vi "Start Sync.vi"(8 "error in (no error)":errorcluster, 11 "gRPC Server in":refnum<class "NiDAQmx.lvclass">) -> (0 "error out":errorcluster, 3 "gRPC Server out":refnum<class "NiDAQmx.lvclass">)   [LabVIEW 2021, in "NI DAQmx_server.lvlib" / "NiDAQmx.lvclass"]
uses:
  NiDAQmx.lvclass
  NiDAQmx.lvclass/NiDAQmx.ctl
  NI DAQmx_wrapper/NI DAQmx_wrapper.lvlib
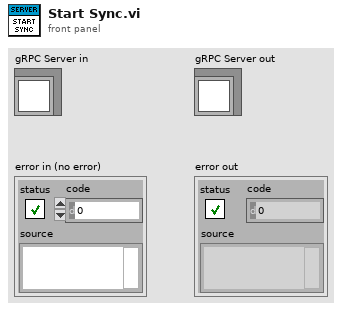
[diagram p1: front panel]
types:
  T1 = typedef "NI DAQmx_server.lvlib/NiDAQmx.lvclass/Server Internal UEs.ctl" = cluster{"NiDAQmx CreateTask Internal UE":refnum<user-event>, "NiDAQmx CreateDOChan Internal UE":refnum<user-event>, "NiDAQmx CreateCIFreqChan Internal UE":refnum<user-event>, "NiDAQmx WriteDigitalLines Internal UE":refnum<user-event>, "NiDAQmx ReadCounterScalarF64 Internal UE":refnum<user-event>, "NiDAQmx CfgImplicitTiming Internal UE":refnum<user-event>, "NiDAQmx StartTask Internal UE":refnum<user-event>, "NiDAQmx StopTask Internal UE":refnum<user-event>, "NiDAQmx ClearTask Internal UE":refnum<user-event>, "NiDAQmx GetTaskAttributeString Internal UE":refnum<user-event>, "NiDAQmx GetChanAttributeString Internal UE":refnum<user-event>, "NiDAQmx GetChanAttributeDouble Internal UE":refnum<user-event>, "NiDAQmx SetChanAttributeString Internal UE":refnum<user-event>, "NiDAQmx SetChanAttributeDouble Internal UE":refnum<user-event>}
  T2 = typedef "NI DAQmx_server.lvlib/NiDAQmx.lvclass/Server gRPC UEs.ctl" = cluster{"NiDAQmx CreateTask gRPC UE":refnum<user-event>, "NiDAQmx CreateDOChan gRPC UE":refnum<user-event>, "NiDAQmx CreateCIFreqChan gRPC UE":refnum<user-event>, "NiDAQmx WriteDigitalLines gRPC UE":refnum<user-event>, "NiDAQmx ReadCounterScalarF64 gRPC UE":refnum<user-event>, "NiDAQmx CfgImplicitTiming gRPC UE":refnum<user-event>, "NiDAQmx StartTask gRPC UE":refnum<user-event>, "NiDAQmx StopTask gRPC UE":refnum<user-event>, "NiDAQmx ClearTask gRPC UE":refnum<user-event>, "NiDAQmx GetTaskAttributeString gRPC UE":refnum<user-event>, "NiDAQmx GetChanAttributeString gRPC UE":refnum<user-event>, "NiDAQmx GetChanAttributeDouble gRPC UE":refnum<user-event>, "NiDAQmx SetChanAttributeString gRPC UE":refnum<user-event>, "NiDAQmx SetChanAttributeDouble gRPC UE":refnum<user-event>}
  T3 = typedef "grpc-lvsupport-release.lvlib/grpcId.ctl" = u64
  T4 = typedef "NI DAQmx_server.lvlib/nidaqmx_grpc_CreateTaskRequest.ctl" = cluster{"session_name":string, "initialization_behavior":T5}
  T5 = typedef "NI DAQmx_server.lvlib/nidevice_grpc_SessionInitializationBehavior.ctl" = enum32{"SESSION_INITIALIZATION_BEHAVIOR_UNSPECIFIED", "SESSION_INITIALIZATION_BEHAVIOR_INITIALIZE_NEW", "SESSION_INITIALIZATION_BEHAVIOR_ATTACH_TO_EXISTING"}
  T6 = typedef "NI DAQmx_server.lvlib/nidaqmx_grpc_CreateTaskResponse.ctl" = cluster{"status":i32, "task":T7, "new_session_initialized":bool}
  T7 = typedef "NI DAQmx_server.lvlib/nidevice_grpc_Session.ctl" = cluster{"nidevice_grpc_Session_session":refnum<class "nidevice_grpc_Session_session.lvclass">}
  T8 = typedef "NI DAQmx_server.lvlib/nidaqmx_grpc_CreateDOChanRequest.ctl" = cluster{"task":T7, "lines":string, "name_to_assign_to_lines":string, "nidaqmx_grpc_CreateDOChanRequest_line_grouping_enum":refnum<class "nidaqmx_grpc_CreateDOChanRequest_line_grouping_enum.lvclass">}
  T9 = typedef "NI DAQmx_server.lvlib/nidaqmx_grpc_CreateDOChanResponse.ctl" = cluster{"status":i32}
  T10 = typedef "NI DAQmx_server.lvlib/nidaqmx_grpc_CreateCIFreqChanRequest.ctl" = cluster{"task":T7, "counter":string, "name_to_assign_to_channel":string, "min_val":dbl, "max_val":dbl, "nidaqmx_grpc_CreateCIFreqChanRequest_units_enum":refnum<class "nidaqmx_grpc_CreateCIFreqChanRequest_units_enum.lvclass">, "nidaqmx_grpc_CreateCIFreqChanRequest_edge_enum":refnum<class "nidaqmx_grpc_CreateCIFreqChanRequest_edge_enum.lvclass">, "nidaqmx_grpc_CreateCIFreqChanRequest_meas_method_enum":refnum<class "nidaqmx_grpc_CreateCIFreqChanRequest_meas_method_enum.lvclass">, "meas_time":dbl, "divisor":u32, "custom_scale_name":string}
  T11 = typedef "NI DAQmx_server.lvlib/nidaqmx_grpc_CreateCIFreqChanResponse.ctl" = cluster{"status":i32}
  T12 = typedef "NI DAQmx_server.lvlib/nidaqmx_grpc_WriteDigitalLinesRequest.ctl" = cluster{"task":T7, "num_samps_per_chan":i32, "auto_start":bool, "timeout":dbl, "nidaqmx_grpc_WriteDigitalLinesRequest_data_layout_enum":refnum<class "nidaqmx_grpc_WriteDigitalLinesRequest_data_layout_enum.lvclass">, "write_array":u8[]}
  T13 = typedef "NI DAQmx_server.lvlib/nidaqmx_grpc_WriteDigitalLinesResponse.ctl" = cluster{"status":i32, "samps_per_chan_written":i32}
  T14 = typedef "NI DAQmx_server.lvlib/nidaqmx_grpc_ReadCounterScalarF64Request.ctl" = cluster{"task":T7, "timeout":dbl}
  T15 = typedef "NI DAQmx_server.lvlib/nidaqmx_grpc_ReadCounterScalarF64Response.ctl" = cluster{"status":i32, "value":dbl}
  T16 = typedef "NI DAQmx_server.lvlib/nidaqmx_grpc_CfgImplicitTimingRequest.ctl" = cluster{"task":T7, "nidaqmx_grpc_CfgImplicitTimingRequest_sample_mode_enum":refnum<class "nidaqmx_grpc_CfgImplicitTimingRequest_sample_mode_enum.lvclass">, "samps_per_chan":u64}
  T17 = typedef "NI DAQmx_server.lvlib/nidaqmx_grpc_CfgImplicitTimingResponse.ctl" = cluster{"status":i32}
  T18 = typedef "NI DAQmx_server.lvlib/nidaqmx_grpc_StartTaskRequest.ctl" = cluster{"task":T7}
  T19 = typedef "NI DAQmx_server.lvlib/nidaqmx_grpc_StartTaskResponse.ctl" = cluster{"status":i32}
  T20 = typedef "NI DAQmx_server.lvlib/nidaqmx_grpc_StopTaskRequest.ctl" = cluster{"task":T7}
  T21 = typedef "NI DAQmx_server.lvlib/nidaqmx_grpc_StopTaskResponse.ctl" = cluster{"status":i32}
  T22 = typedef "NI DAQmx_server.lvlib/nidaqmx_grpc_ClearTaskRequest.ctl" = cluster{"task":T7}
  T23 = typedef "NI DAQmx_server.lvlib/nidaqmx_grpc_ClearTaskResponse.ctl" = cluster{"status":i32}
  T24 = typedef "NI DAQmx_server.lvlib/nidaqmx_grpc_GetTaskAttributeStringRequest.ctl" = cluster{"task":T7, "nidaqmx_grpc_GetTaskAttributeStringRequest_attribute_enum":refnum<class "nidaqmx_grpc_GetTaskAttributeStringRequest_attribute_enum.lvclass">}
  T25 = typedef "NI DAQmx_server.lvlib/nidaqmx_grpc_GetTaskAttributeStringResponse.ctl" = cluster{"status":i32, "value":string}
  T26 = typedef "NI DAQmx_server.lvlib/nidaqmx_grpc_GetChanAttributeStringRequest.ctl" = cluster{"task":T7, "channel":string, "nidaqmx_grpc_GetChanAttributeStringRequest_attribute_enum":refnum<class "nidaqmx_grpc_GetChanAttributeStringRequest_attribute_enum.lvclass">}
  T27 = typedef "NI DAQmx_server.lvlib/nidaqmx_grpc_GetChanAttributeStringResponse.ctl" = cluster{"status":i32, "value":string}
  T28 = typedef "NI DAQmx_server.lvlib/nidaqmx_grpc_GetChanAttributeDoubleRequest.ctl" = cluster{"task":T7, "channel":string, "nidaqmx_grpc_GetChanAttributeDoubleRequest_attribute_enum":refnum<class "nidaqmx_grpc_GetChanAttributeDoubleRequest_attribute_enum.lvclass">}
  T29 = typedef "NI DAQmx_server.lvlib/nidaqmx_grpc_GetChanAttributeDoubleResponse.ctl" = cluster{"status":i32, "value":dbl}
  T30 = typedef "NI DAQmx_server.lvlib/nidaqmx_grpc_SetChanAttributeStringRequest.ctl" = cluster{"task":T7, "channel":string, "nidaqmx_grpc_SetChanAttributeStringRequest_attribute_enum":refnum<class "nidaqmx_grpc_SetChanAttributeStringRequest_attribute_enum.lvclass">, "value":string}
  T31 = typedef "NI DAQmx_server.lvlib/nidaqmx_grpc_SetChanAttributeStringResponse.ctl" = cluster{"status":i32}
  T32 = typedef "NI DAQmx_server.lvlib/nidaqmx_grpc_SetChanAttributeDoubleRequest.ctl" = cluster{"task":T7, "channel":string, "nidaqmx_grpc_SetChanAttributeDoubleRequest_attribute_enum":refnum<class "nidaqmx_grpc_SetChanAttributeDoubleRequest_attribute_enum.lvclass">, "value":dbl}
  T33 = typedef "NI DAQmx_server.lvlib/nidaqmx_grpc_SetChanAttributeDoubleResponse.ctl" = cluster{"status":i32}
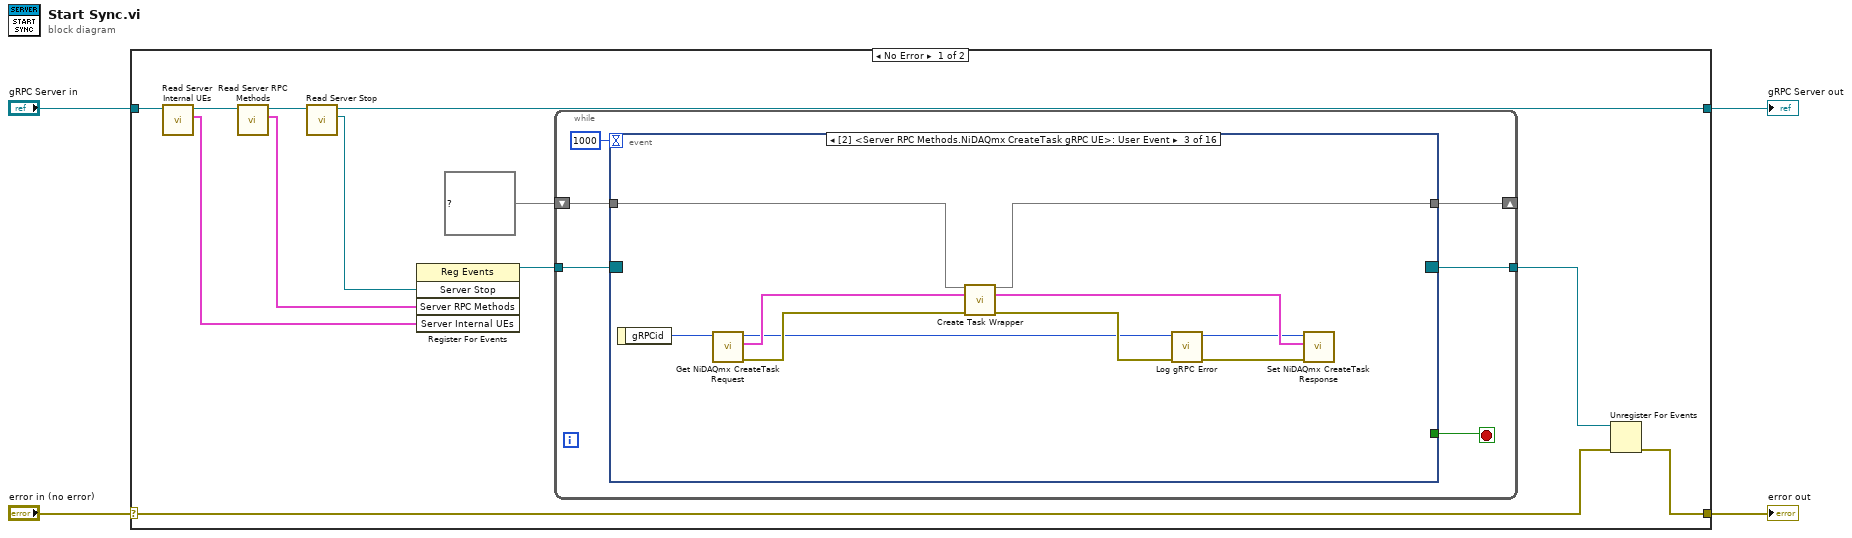
[diagram p0: block diagram]
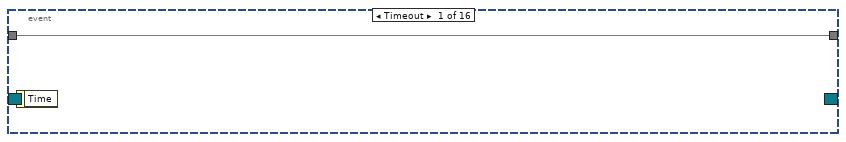
[diagram p2: hidden frame]
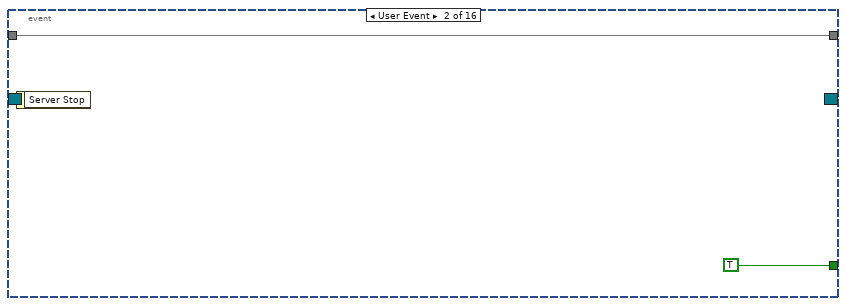
[diagram p3: hidden frame]
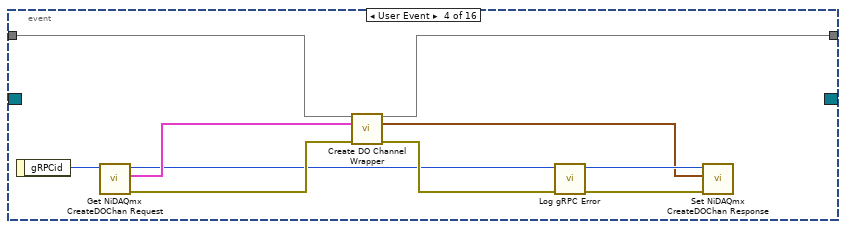
[diagram p4: hidden frame]
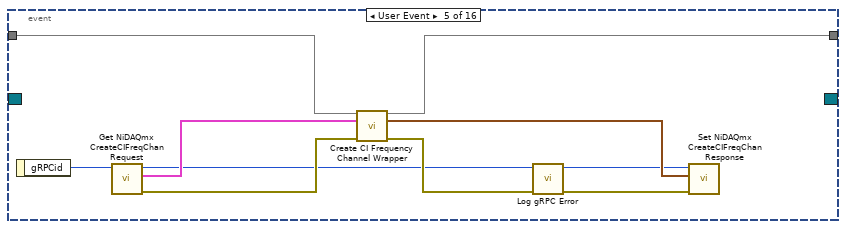
[diagram p5: hidden frame]
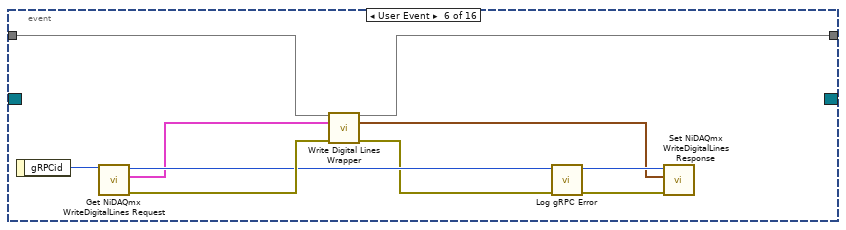
[diagram p6: hidden frame]
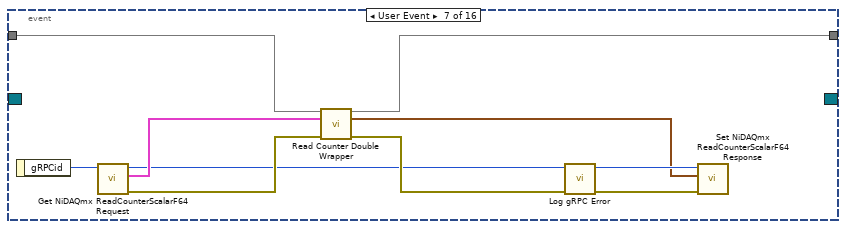
[diagram p7: hidden frame]
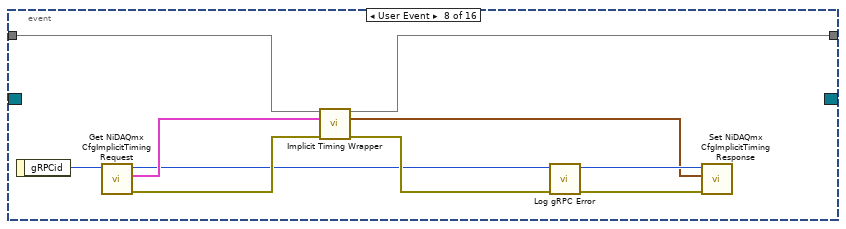
[diagram p8: hidden frame]
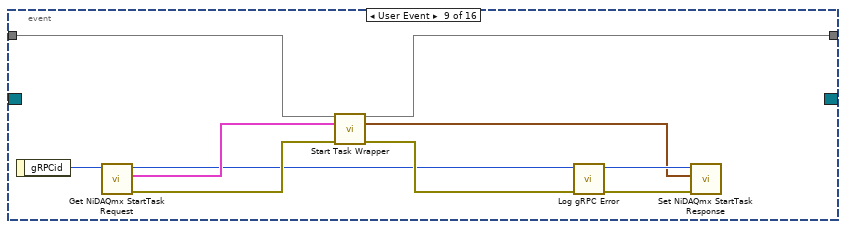
[diagram p9: hidden frame]
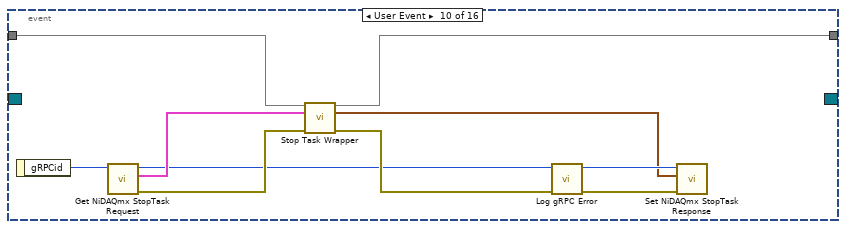
[diagram p10: hidden frame]
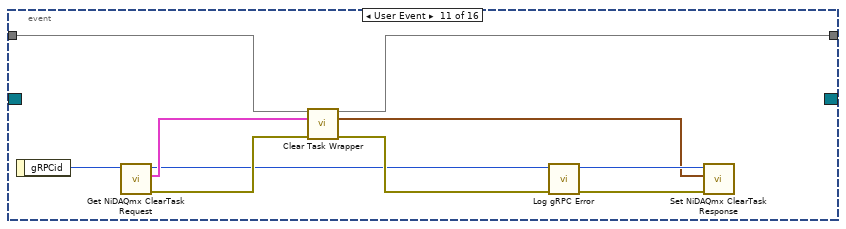
[diagram p11: hidden frame]
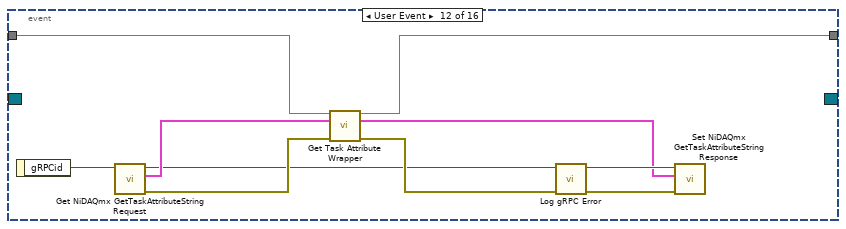
[diagram p12: hidden frame]
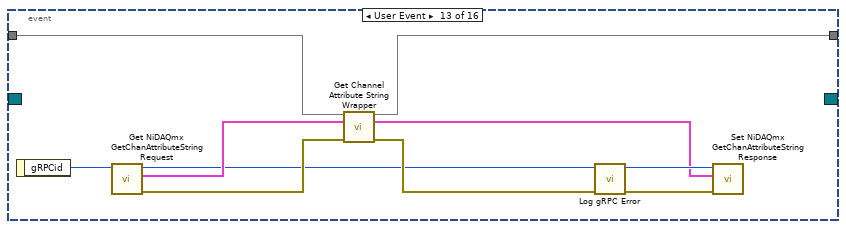
[diagram p13: hidden frame]
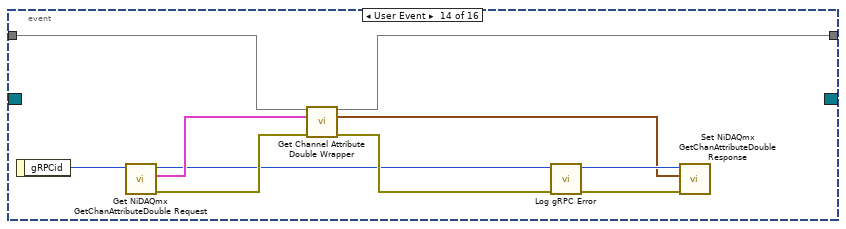
[diagram p14: hidden frame]
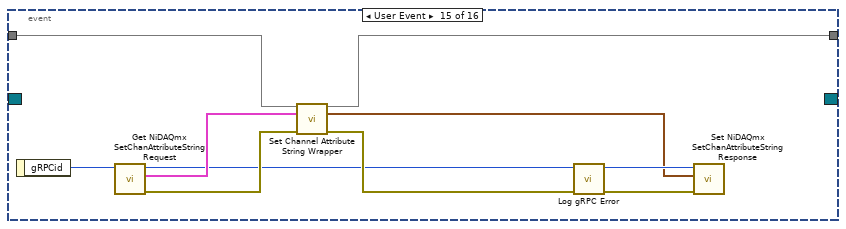
[diagram p15: hidden frame]
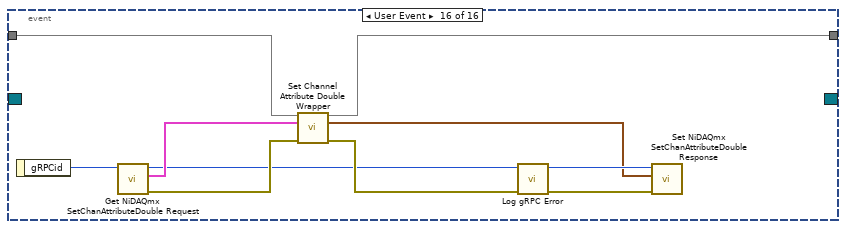
[diagram p16: hidden frame]
diagram:
  n1 = case shown="No Error" "error in (no error)" {
    selector: "error in (no error)" -> [w10 w167]
    tunnel: [w9 w167] -> w3
    tunnel: [w7 w166] -> w1
    tunnel: "gRPC Server in" -> [w16 w166]
    frame No Error {
      n2 = call "Read Server Internal UEs.vi"("SignalGeneratorService in"=w16) -> ("Server Internal UEs"=w14:T1, "SignalGeneratorService out"=w15:refnum<class "NiDAQmx.lvclass">)  [unwired: 8 in, 1 out]
      n3 = call "Read Server RPC Methods.vi"("SignalGeneratorService in"=w15) -> ("Server RPC Methods"=w8:T2, "SignalGeneratorService out"=w13:refnum<class "NiDAQmx.lvclass">)  [unwired: 8 in, 1 out]
      n4 = call-dynamic "Read Server Stop.vi"("iService in"=w13) -> ("Server Stop"=w6:refnum<user-event>, "iService out"=w7:refnum<class "NiDAQmx.lvclass">)  [unwired: 8 in, 1 out]
      n5 = register-events(w6, w8, w14) -> (reference out=w12:refnum<event-registration>)  [unwired: 2 in, 1 out]
      n6 = while {
        tunnel: w12 -> [w22]
        tunnel: [w20] -> w11
        shift-right: [w17] -> _
        shift-left: map{string, refnum<k21>} {} ("Task map") -> [w18]
        stop <- w21 stop-if-true
        n7 = event "RPC Methods Event Structure" shown="[2] <Server RPC Methods.NiDAQmx CreateTask gRPC UE>: User Event" {
          selector: w22 -> [_ _ _ _ _ _ _ _ _ _ _ _ _ _ _ _]
          dyn-events: [_ _ _ _ _ _ _ _ _ _ _ _ _ _ _ _] -> w20
          timeout: 1000 -> [_ _ _ _ _ _ _ _ _ _ _ _ _ _ _ _]
          tunnel: [_ TRUE _ _ _ _ _ _ _ _ _ _ _ _ _ _] -> w21
          tunnel: w18 -> [w23 w24 w32 w42 w47 w60 w73 w82 w92 w102 w113 w123 w132 w142 w152 w162]
          tunnel: [w23 w24 w30 w36 w46 w58 w71 w77 w91 w100 w107 w116 w127 w137 w150 w157] -> w17
          event Timeout {
            n8 = event-data() -> ()  [unwired: 1 in, 1 out]
          }
          event User Event {
            n9 = event-data() -> ()  [unwired: 1 in, 1 out]
          }
          event User Event {
            n10 = event-data() -> ("gRPCid"=w35:T3)  [unwired: 1 in]
            n11 = call "Get NiDAQmx CreateTask Request.vi"("gRPCid"=w35) -> ("error out"=w34:errorcluster, "Message Data"=w33:T4, "gRPCid out"=w27:T3)  [unwired: 8 in]
            n12 = call "Create Task Wrapper.vi"("Task map in"=w32, "Message Data in"=w33, "error in (no error)"=w34) -> ("Task map out"=w30:map{string, refnum<k21>}, "Message Data out"=w31:T6, "error out"=w29:errorcluster)  [unwired: 10 in]
            n13 = call "Log gRPC Error.vi"("error IO"=w29, "gRPC ID in"=w27) -> ("error out"=w28:errorcluster, "gRPCid out"=w26:T3)  [unwired: 8 in]
            n14 = call "Set NiDAQmx CreateTask Response.vi"("error in (no error)"=w28, "Message Data"=w31, "gRPCid in"=w26) -> ()  [unwired: 8 in, 1 out]
          }
          event User Event {
            n15 = event-data() -> ("gRPCid"=w45:T3)  [unwired: 1 in]
            n16 = call "Get NiDAQmx CreateDOChan Request.vi"("gRPCid"=w45) -> ("error out"=w44:errorcluster, "Message Data"=w43:T8, "gRPCid out"=w39:T3)  [unwired: 8 in]
            n17 = call "Create DO Channel Wrapper.vi"("Task map in"=w42, "Message Data in"=w43, "error in (no error)"=w44) -> ("Task map out"=w36:map{string, refnum<k21>}, "Message Data out"=w37:T9, "error out"=w41:errorcluster)  [unwired: 10 in]
            n18 = call "Log gRPC Error.vi"("error IO"=w41, "gRPC ID in"=w39) -> ("error out"=w40:errorcluster, "gRPCid out"=w38:T3)  [unwired: 8 in]
            n19 = call "Set NiDAQmx CreateDOChan Response.vi"("error in (no error)"=w40, "Message Data"=w37, "gRPCid in"=w38) -> ()  [unwired: 8 in, 1 out]
          }
          event User Event {
            n20 = event-data() -> ("gRPCid"=w55:T3)  [unwired: 1 in]
            n21 = call "Get NiDAQmx CreateCIFreqChan Request.vi"("gRPCid"=w55) -> ("error out"=w54:errorcluster, "Message Data"=w53:T10, "gRPCid out"=w49:T3)  [unwired: 8 in]
            n22 = call "Create CI Frequency Channel Wrapper.vi"("Task map in"=w47, "Message Data in"=w53, "error in (no error)"=w54) -> ("Task map out"=w46:map{string, refnum<k21>}, "Message Data out"=w50:T11, "error out"=w51:errorcluster)  [unwired: 10 in]
            n23 = call "Log gRPC Error.vi"("error IO"=w51, "gRPC ID in"=w49) -> ("error out"=w52:errorcluster, "gRPCid out"=w48:T3)  [unwired: 8 in]
            n24 = call "Set NiDAQmx CreateCIFreqChan Response.vi"("error in (no error)"=w52, "Message Data"=w50, "gRPCid in"=w48) -> ()  [unwired: 8 in, 1 out]
          }
          event User Event {
            n25 = event-data() -> ("gRPCid"=w65:T3)  [unwired: 1 in]
            n26 = call "Get NiDAQmx WriteDigitalLines Request.vi"("gRPCid"=w65) -> ("error out"=w64:errorcluster, "Message Data"=w59:T12, "gRPCid out"=w62:T3)  [unwired: 8 in]
            n27 = call "Write Digital Lines Wrapper.vi"("Task map in"=w60, "Message Data in"=w59, "error in (no error)"=w64) -> ("Task map out"=w58:map{string, refnum<k21>}, "Message Data out"=w57:T13, "error out"=w56:errorcluster)  [unwired: 10 in]
            n28 = call "Log gRPC Error.vi"("error IO"=w56, "gRPC ID in"=w62) -> ("error out"=w63:errorcluster, "gRPCid out"=w61:T3)  [unwired: 8 in]
            n29 = call "Set NiDAQmx WriteDigitalLines Response.vi"("error in (no error)"=w63, "Message Data"=w57, "gRPCid in"=w61) -> ()  [unwired: 8 in, 1 out]
          }
          event User Event {
            n30 = event-data() -> ("gRPCid"=w75:T3)  [unwired: 1 in]
            n31 = call "Get NiDAQmx ReadCounterScalarF64 Request.vi"("gRPCid"=w75) -> ("error out"=w74:errorcluster, "Message Data"=w72:T14, "gRPCid out"=w68:T3)  [unwired: 8 in]
            n32 = call "Read Counter Double Wrapper.vi"("Task map in"=w73, "Message Data in"=w72, "error in (no error)"=w74) -> ("Task map out"=w71:map{string, refnum<k21>}, "Message Data Out"=w66:T15, "error out"=w70:errorcluster)  [unwired: 10 in]
            n33 = call "Log gRPC Error.vi"("error IO"=w70, "gRPC ID in"=w68) -> ("error out"=w69:errorcluster, "gRPCid out"=w67:T3)  [unwired: 8 in]
            n34 = call "Set NiDAQmx ReadCounterScalarF64 Response.vi"("error in (no error)"=w69, "Message Data"=w66, "gRPCid in"=w67) -> ()  [unwired: 8 in, 1 out]
          }
          event User Event {
            n35 = event-data() -> ("gRPCid"=w85:T3)  [unwired: 1 in]
            n36 = call "Get NiDAQmx CfgImplicitTiming Request.vi"("gRPCid"=w85) -> ("error out"=w84:errorcluster, "Message Data"=w83:T16, "gRPCid out"=w79:T3)  [unwired: 8 in]
            n37 = call "Implicit Timing Wrapper.vi"("Task map in"=w82, "Message Data in"=w83, "error in (no error)"=w84) -> ("Task map out"=w77:map{string, refnum<k21>}, "Message Data out"=w76:T17, "error out"=w81:errorcluster)  [unwired: 10 in]
            n38 = call "Log gRPC Error.vi"("error IO"=w81, "gRPC ID in"=w79) -> ("error out"=w80:errorcluster, "gRPCid out"=w78:T3)  [unwired: 8 in]
            n39 = call "Set NiDAQmx CfgImplicitTiming Response.vi"("error in (no error)"=w80, "Message Data"=w76, "gRPCid in"=w78) -> ()  [unwired: 8 in, 1 out]
          }
          event User Event {
            n40 = event-data() -> ("gRPCid"=w95:T3)  [unwired: 1 in]
            n41 = call "Get NiDAQmx StartTask Request.vi"("gRPCid"=w95) -> ("error out"=w94:errorcluster, "Message Data"=w93:T18, "gRPCid out"=w88:T3)  [unwired: 8 in]
            n42 = call "Start Task Wrapper.vi"("Task map in"=w92, "Message Data in"=w93, "error in (no error)"=w94) -> ("Task map out"=w91:map{string, refnum<k21>}, "Message Data out"=w86:T19, "error out"=w90:errorcluster)  [unwired: 10 in]
            n43 = call "Log gRPC Error.vi"("error IO"=w90, "gRPC ID in"=w88) -> ("error out"=w89:errorcluster, "gRPCid out"=w87:T3)  [unwired: 8 in]
            n44 = call "Set NiDAQmx StartTask Response.vi"("error in (no error)"=w89, "Message Data"=w86, "gRPCid in"=w87) -> ()  [unwired: 8 in, 1 out]
          }
          event User Event {
            n45 = event-data() -> ("gRPCid"=w105:T3)  [unwired: 1 in]
            n46 = call "Get NiDAQmx StopTask Request.vi"("gRPCid"=w105) -> ("error out"=w104:errorcluster, "Message Data"=w103:T20, "gRPCid out"=w98:T3)  [unwired: 8 in]
            n47 = call "Stop Task Wrapper.vi"("Task map in"=w102, "Message Data in"=w103, "error in (no error)"=w104) -> ("Task map out"=w100:map{string, refnum<k21>}, "Message Data out"=w96:T21, "error out"=w101:errorcluster)  [unwired: 10 in]
            n48 = call "Log gRPC Error.vi"("error IO"=w101, "gRPC ID in"=w98) -> ("error out"=w99:errorcluster, "gRPCid out"=w97:T3)  [unwired: 8 in]
            n49 = call "Set NiDAQmx StopTask Response.vi"("error in (no error)"=w99, "Message Data"=w96, "gRPCid in"=w97) -> ()  [unwired: 8 in, 1 out]
          }
          event User Event {
            n50 = event-data() -> ("gRPCid"=w115:T3)  [unwired: 1 in]
            n51 = call "Get NiDAQmx ClearTask Request.vi"("gRPCid"=w115) -> ("error out"=w114:errorcluster, "Message Data"=w112:T22, "gRPCid out"=w109:T3)  [unwired: 8 in]
            n52 = call "Clear Task Wrapper.vi"("Task map in"=w113, "Message Data in"=w112, "error in (no error)"=w114) -> ("Task map out"=w107:map{string, refnum<k21>}, "Message Data out"=w106:T23, "error out"=w111:errorcluster)  [unwired: 10 in]
            n53 = call "Log gRPC Error.vi"("error IO"=w111, "gRPC ID in"=w109) -> ("error out"=w110:errorcluster, "gRPCid out"=w108:T3)  [unwired: 8 in]
            n54 = call "Set NiDAQmx ClearTask Response.vi"("error in (no error)"=w110, "Message Data"=w106, "gRPCid in"=w108) -> ()  [unwired: 8 in, 1 out]
          }
          event User Event {
            n55 = event-data() -> ("gRPCid"=w125:T3)  [unwired: 1 in]
            n56 = call "Get NiDAQmx GetTaskAttributeString Request.vi"("gRPCid"=w125) -> ("error out"=w124:errorcluster, "Message Data"=w122:T24, "gRPCid out"=w119:T3)  [unwired: 8 in]
            n57 = call "Get Task Attribute Wrapper.vi"("Task map in"=w123, "Message Data in"=w122, "error in (no error)"=w124) -> ("Task map out"=w116:map{string, refnum<k21>}, "Message Data out"=w117:T25, "error out"=w121:errorcluster)  [unwired: 10 in]
            n58 = call "Log gRPC Error.vi"("error IO"=w121, "gRPC ID in"=w119) -> ("error out"=w120:errorcluster, "gRPCid out"=w118:T3)  [unwired: 8 in]
            n59 = call "Set NiDAQmx GetTaskAttributeString Response.vi"("error in (no error)"=w120, "Message Data"=w117, "gRPCid in"=w118) -> ()  [unwired: 8 in, 1 out]
          }
          event User Event {
            n60 = event-data() -> ("gRPCid"=w135:T3)  [unwired: 1 in]
            n61 = call "Get NiDAQmx GetChanAttributeString Request.vi"("gRPCid"=w135) -> ("error out"=w134:errorcluster, "Message Data"=w133:T26, "gRPCid out"=w129:T3)  [unwired: 8 in]
            n62 = call "Get Channel Attribute String Wrapper.vi"("Task map in"=w132, "Message Data in"=w133, "error in (no error)"=w134) -> ("Task map out"=w127:map{string, refnum<k21>}, "Message Data out"=w126:T27, "error out"=w131:errorcluster)  [unwired: 10 in]
            n63 = call "Log gRPC Error.vi"("error IO"=w131, "gRPC ID in"=w129) -> ("error out"=w130:errorcluster, "gRPCid out"=w128:T3)  [unwired: 8 in]
            n64 = call "Set NiDAQmx GetChanAttributeString Response.vi"("error in (no error)"=w130, "Message Data"=w126, "gRPCid in"=w128) -> ()  [unwired: 8 in, 1 out]
          }
          event User Event {
            n65 = event-data() -> ("gRPCid"=w145:T3)  [unwired: 1 in]
            n66 = call "Get NiDAQmx GetChanAttributeDouble Request.vi"("gRPCid"=w145) -> ("error out"=w144:errorcluster, "Message Data"=w143:T28, "gRPCid out"=w139:T3)  [unwired: 8 in]
            n67 = call "Get Channel Attribute Double Wrapper.vi"("Task map in"=w142, "Message Data in"=w143, "error in (no error)"=w144) -> ("Task map out"=w137:map{string, refnum<k21>}, "Message Data out"=w136:T29, "error out"=w141:errorcluster)  [unwired: 10 in]
            n68 = call "Log gRPC Error.vi"("error IO"=w141, "gRPC ID in"=w139) -> ("error out"=w140:errorcluster, "gRPCid out"=w138:T3)  [unwired: 8 in]
            n69 = call "Set NiDAQmx GetChanAttributeDouble Response.vi"("error in (no error)"=w140, "Message Data"=w136, "gRPCid in"=w138) -> ()  [unwired: 8 in, 1 out]
          }
          event User Event {
            n70 = event-data() -> ("gRPCid"=w155:T3)  [unwired: 1 in]
            n71 = call "Get NiDAQmx SetChanAttributeString Request.vi"("gRPCid"=w155) -> ("error out"=w154:errorcluster, "Message Data"=w153:T30, "gRPCid out"=w148:T3)  [unwired: 8 in]
            n72 = call "Set Channel Attribute String Wrapper.vi"("Task map in"=w152, "Message Data in"=w153, "error in (no error)"=w154) -> ("Task map out"=w150:map{string, refnum<k21>}, "Message Data out"=w146:T31, "error out"=w151:errorcluster)  [unwired: 10 in]
            n73 = call "Log gRPC Error.vi"("error IO"=w151, "gRPC ID in"=w148) -> ("error out"=w149:errorcluster, "gRPCid out"=w147:T3)  [unwired: 8 in]
            n74 = call "Set NiDAQmx SetChanAttributeString Response.vi"("error in (no error)"=w149, "Message Data"=w146, "gRPCid in"=w147) -> ()  [unwired: 8 in, 1 out]
          }
          event User Event {
            n75 = event-data() -> ("gRPCid"=w165:T3)  [unwired: 1 in]
            n76 = call "Get NiDAQmx SetChanAttributeDouble Request.vi"("gRPCid"=w165) -> ("error out"=w164:errorcluster, "Message Data"=w163:T32, "gRPCid out"=w159:T3)  [unwired: 8 in]
            n77 = call "Set Channel Attribute Double Wrapper.vi"("Task map in"=w162, "Message Data in"=w163, "error in (no error)"=w164) -> ("Task map out"=w157:map{string, refnum<k21>}, "Message Data out"=w156:T33, "error out"=w161:errorcluster)  [unwired: 10 in]
            n78 = call "Log gRPC Error.vi"("error IO"=w161, "gRPC ID in"=w159) -> ("error out"=w160:errorcluster, "gRPCid out"=w158:T3)  [unwired: 8 in]
            n79 = call "Set NiDAQmx SetChanAttributeDouble Response.vi"("error in (no error)"=w160, "Message Data"=w156, "gRPCid in"=w158) -> ()  [unwired: 8 in, 1 out]
          }
        }
      }
      n80 = Unregister For Events(event registration refnum=w11, error in=w10) -> (error out=w9:errorcluster)
    }
    frame Error {
    }
  }
  "error out" <- w3
  "gRPC Server out" <- w1
